vi "LED color changer.vi"(0 "MASTER":dbl=1.0 min=1.0 max=10.0 step=1.0, 1 "IP":string="192.168.23.100", 2 "Function":enum16{"READ", "Write"}(ring), 5 "PORT":dbl=1.0 min=1.0 max=4.0 step=1.0, 7 "ON/OFF / ALARM":enum16{"ON", "OFF", "ALARM"}(ring), 9 "Color select":T1(ring), 11 "error in (no error)":errorcluster) -> (4 "Color":bool, 6 "Colors [4]":cluster{u32, u32}[](array[cluster]), 15 "error out":errorcluster)   [LabVIEW 2022 SP3]
uses:
  <vilib>/NI/Advanced HTTP Client/POST (Buffer).vi
  <vilib>/NI/Advanced HTTP Client/Session.lvclass
  <vilib>/JDP Science/JSONtext/JSONtext.lvlib
panel:
  # "Parameter Query"
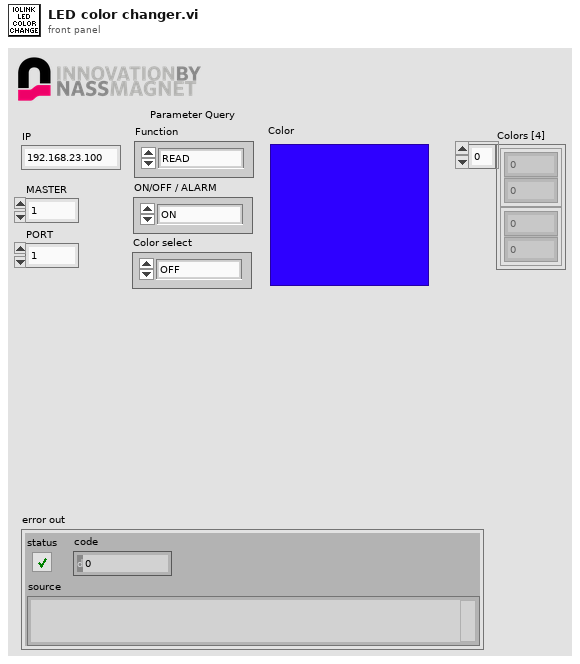
[diagram p1: front panel]
types:
  T1 = enum16{"OFF", "Blue", "Green", "Cyan", "Red", "Magenta", "Yellow", "White", ""}
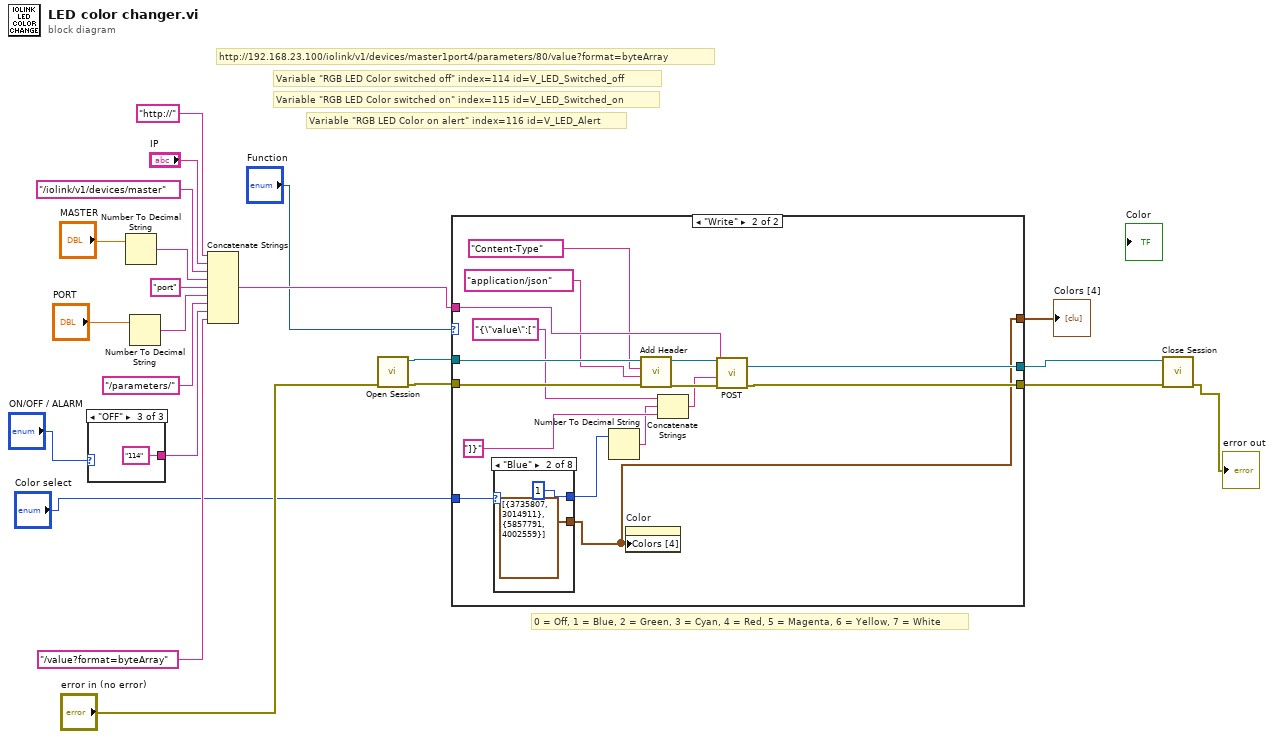
[diagram p0: block diagram]
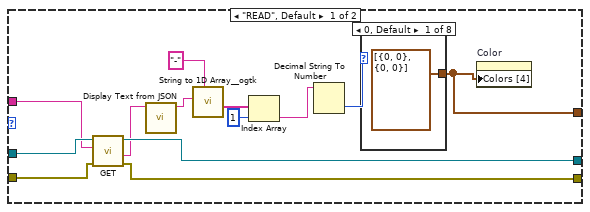
[diagram p2: hidden frame]
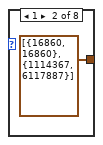
[diagram p3: hidden frame]
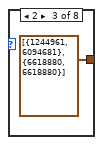
[diagram p4: hidden frame]
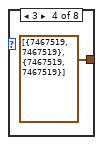
[diagram p5: hidden frame]
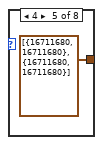
[diagram p6: hidden frame]
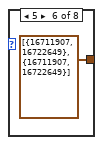
[diagram p7: hidden frame]
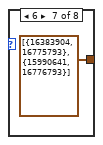
[diagram p8: hidden frame]
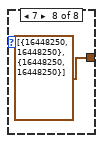
[diagram p9: hidden frame]
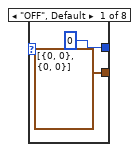
[diagram p10: hidden frame]
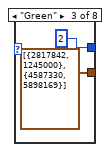
[diagram p11: hidden frame]
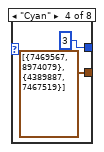
[diagram p12: hidden frame]
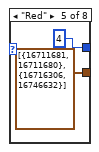
[diagram p13: hidden frame]
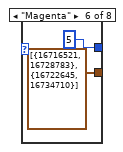
[diagram p14: hidden frame]
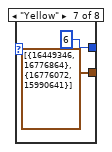
[diagram p15: hidden frame]
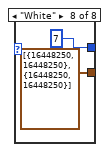
[diagram p16: hidden frame]
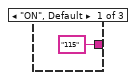
[diagram p17: hidden frame]
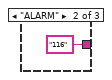
[diagram p18: hidden frame]
diagram:
  # "0 = Off, 1 = Blue, 2 = Green, 3 = Cyan, 4 = Red, 5 = Magenta, 6 = Yellow, 7 = White"
  # "Variable \"RGB LED Color on alert\" index=116 id=V_LED_Alert"
  # "Variable \"RGB LED Color switched on\" index=115 id=V_LED_Switched_on"
  # "Variable \"RGB LED Color switched off\" index=114 id=V_LED_Switched_off"
  # "http://192.168.23.100/iolink/v1/devices/master1port4/parameters/80/value?format=byteArray"
  n1 = case shown="\"OFF\"" "ON/OFF / ALARM" {
    tunnel: ["115" ("PARAMETERS") "116" ("PARAMETERS") "114" ("PARAMETERS")] -> w14
    frame "ON", Default {
    }
    frame "ALARM" {
    }
    frame "OFF" {
    }
  }
  n2 = Number To Decimal String(number="MASTER") -> (decimal integer string=w11:string)  [unwired: 1 in]
  n3 = Number To Decimal String(number="PORT") -> (decimal integer string=w8:string)  [unwired: 1 in]
  n4 = Concatenate Strings("http://" ("string"), "IP", "/iolink/v1/devices/master" ("string"), w11, "port" ("string"), w8, "/parameters/" ("string"), w14, "/value?format=byteArray" ("string")) -> (w12:string)
  n5 = call <vilib>:"Open Session.vi"("error in"="error in (no error)") -> ("error out"=w21:errorcluster, "session"=w22:refnum<class "Session.lvclass">)  [unwired: 9 in]
  n6 = case shown="\"Write\"" "Function" {
    tunnel: w22 -> [w37 w58]
    tunnel: w21 -> [w36 w59]
    tunnel: w12 -> [w34 w62]
    tunnel: [w38 w61] -> w7
    tunnel: [w35 w60] -> w6
    tunnel: "Color select" -> [_ w49]
    tunnel: [w26 w47] -> w1
    frame "READ", Default {
      n7 = call <vilib>:"GET.vi"("error in"=w36, "url"=w34, "session in"=w37) -> ("error out"=w35:errorcluster, "body"=w33:string, "session out"=w38:refnum<class "Session.lvclass">)  [unwired: 4 in, 2 out]
      n8 = call <vilib>:"Display Text from JSON.vi"("Input JSON"=w33) -> ("Display Text"=w32:string)  [unwired: 8 in, 2 out]
      n9 = call <userlib>:"String to 1D Array__ogtk.vi"("delimiter (Tab)"="-", "string"=w32) -> ("Array of Strings"=w30:string[])  [unwired: 9 in]
      n10 = Index Array(array=w30, index=1) -> (element=w28:string)
      n11 = Decimal String To Number(string=w28) -> (number=w27:i32)  [unwired: 2 in, 1 out]
      n12 = case shown="0, Default" w27 {
        tunnel: [cluster{u32, u32}[] [{0, 0}, {0, 0}] ("Colors [4]") cluster{u32, u32}[] [{16860, 16860}, {1114367, 6117887}] ("Colors [4]") cluster{u32, u32}[] [{1244961, 6094681}, {6618880, 6618880}] ("Colors [4]") cluster{u32, u32}[] [{7467519, 7467519}, {7467519, 7467519}] ("Colors [4]") cluster{u32, u32}[] [{16711680, 16711680}, {16711680, 16711680}] ("Colors [4]") cluster{u32, u32}[] [{16711907, 16722649}, {16711907, 16722649}] ("Colors [4]") cluster{u32, u32}[] [{16383904, 16775793}, {15990641, 16776793}] ("Colors [4]") cluster{u32, u32}[] [{16448250, 16448250}, {16448250, 16448250}] ("Colors [4]")] -> w26
        frame 0, Default {
        }
        frame 1 {
        }
        frame 2 {
        }
        frame 3 {
        }
        frame 4 {
        }
        frame 5 {
        }
        frame 6 {
        }
        frame 7 {
        }
      }
      n13 = property on="Color" class="Bool (strict)"("Colors [4]"=w26) -> ()  [unwired: 2 in, 2 out]
    }
    frame "Write" {
      n14 = case shown="\"Blue\"" w49 {
        tunnel: [0 1 2 3 4 5 6 7] -> w48
        tunnel: [cluster{u32, u32}[] [{0, 0}, {0, 0}] ("Colors [4]") cluster{u32, u32}[] [{3735807, 3014911}, {5857791, 4002559}] ("Colors [4]") cluster{u32, u32}[] [{2817842, 1245000}, {4587330, 5898169}] ("Colors [4]") cluster{u32, u32}[] [{7469567, 8974079}, {4389887, 7467519}] ("Colors [4]") cluster{u32, u32}[] [{16711681, 16711680}, {16716306, 16746632}] ("Colors [4]") cluster{u32, u32}[] [{16716521, 16728783}, {16722645, 16734710}] ("Colors [4]") cluster{u32, u32}[] [{16449346, 16776864}, {16776072, 15990641}] ("Colors [4]") cluster{u32, u32}[] [{16448250, 16448250}, {16448250, 16448250}] ("Colors [4]")] -> w47
        frame "OFF", Default {
        }
        frame "Blue" {
        }
        frame "Green" {
        }
        frame "Cyan" {
        }
        frame "Red" {
        }
        frame "Magenta" {
        }
        frame "Yellow" {
        }
        frame "White" {
        }
      }
      n15 = Number To Decimal String(number=w48) -> (decimal integer string=w50:string)  [unwired: 1 in]
      n16 = property on="Color" class="Bool (strict)"("Colors [4]"=w47) -> ()  [unwired: 2 in, 2 out]
      n17 = call <vilib>:"Add Header.vi"("error in"=w59, "value"="application/json" ("buffer"), "header"="Content-Type", "session in"=w58) -> ("error out"=w56:errorcluster, "session out"=w57:refnum<class "Session.lvclass">)  [unwired: 6 in]
      n18 = Concatenate Strings("{\"value\":[" ("buffer"), w50, "]}" ("string")) -> (w53:string)
      n19 = call-poly <vilib>:"POST.vi"("error in"=w56, "buffer"=w53, "url"=w62, "session in"=w57) -> ("error out"=w60:errorcluster, "session out"=w61:refnum<class "Session.lvclass">)  [unwired: 3 in, 3 out]
    }
  }
  "Colors [4]" <- w1
  n20 = call <vilib>:"Close Session.vi"("error in"=w6, "session"=w7) -> ("error out"=→"error out":errorcluster)  [unwired: 9 in]
